vi "CgDataCollect.vi"(0 "Data Queue":refnum<queue>, 1 "Timed Structure Name":string, 2 "Timing Source":string="1 kHz", 5 "VISA resource name":refnum<visa-resource-name>, 7 "Bytes to Read":i32, 9 "Relative Time":u32, 11 "error in (no error)":errorcluster, 12 "Time Loop Priority":i32=100, 13 "Time Bytes Before Output":i16) -> (4 "Queue Out":refnum<queue>, 6 "VISA resource name out":refnum<visa-resource-name>, 8 "Timing Array":u32[](array[numeric]), 15 "error out":errorcluster)   [LabVIEW 2012]
doc: "Collects data from the cyberglove.\nQueries the cyberglove for data and sends the data to a queue to be read by an interpreter running in parallel. Using the relative time and the time bytes before output causes the program to put a time stamp in ms before the output."
uses:
  <vilib>/Platform/TimedLoop/XDataNode/timing_clust.ctl
  <vilib>/Platform/TimedLoop/XDataNode/nitl_modes.ctl
  <vilib>/Platform/TimedLoop/XDataNode/wakeup.ctl
  GlobalVariables.vi
  <vilib>/Platform/TimedLoop/XDataNode/XDataNode.xnode
  <vilib>/Platform/TimedLoop/XDataNode/XDNodeRunTimeDep.lvlib
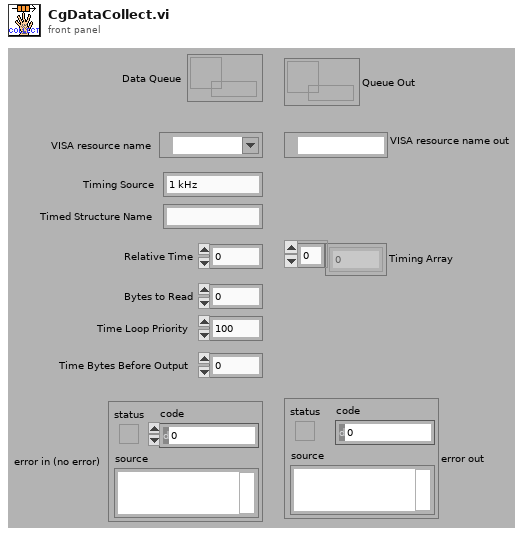
[diagram p1: front panel]
types:
  T1 = typedef "XDNodeRunTimeDep.lvlib/timing_clust.ctl" = cluster{"Expected End [f-1]":u64, "Actual End [f-1]":u64, "Finished Late? [f-1]":bool, "Expected End [i-1]":u64, "Actual End [i-1]":u64, "Finished Late? [i-1]":bool, "Expected Start [i]":u64, "Actual Start [i]":u64, "Expected Start [f]":u64, "Actual Start [f]":u64, "Source Name":string, "Structure Name":string, "Period":i64, "Deadline":i64, "Offset":i64, "Start":i64, "Priority":i32, "Timeout":i32, "Mode":T2, "Wakeup Reason":T3, "Error":errorcluster, "Source Type":string, "Secondary Source Type":string, "Global End Time":u64, "Global Start Time":u64, "Frame Duration":u64, "Iteration Duration":u64, "Assigned CPU":i32, "I/O Scan Engine Mode":u32}
  T2 = typedef "XDNodeRunTimeDep.lvlib/nitl_modes.ctl" = enum32{"No Change", "Process missed periods, maintain original phase", "Discard missed periods, maintain original phase", "Process missed periods, ignore original phase", "Discard missed periods, ignore original phase"}
  T3 = typedef "XDNodeRunTimeDep.lvlib/wakeup.ctl" = enum32{"Normal", "Aborted", "Asynchronous wakeup", "Timing source error", "Timed loop error", "Timeout"}
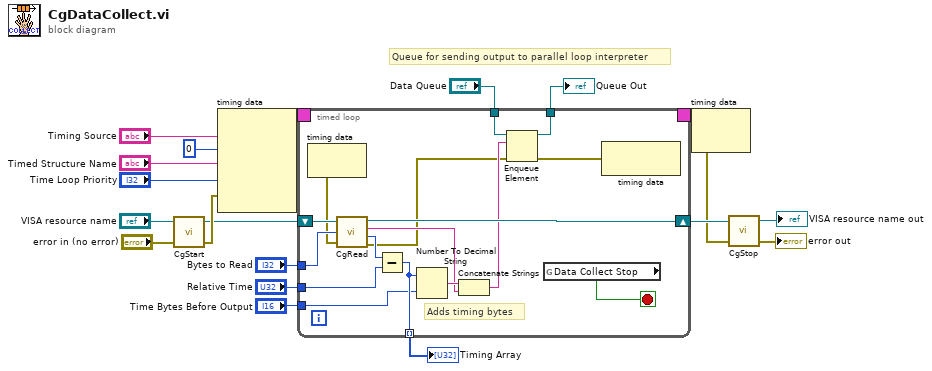
[diagram p0: block diagram]
diagram:
  # "Queue for sending output to parallel loop interpreter"
  n1 = call "CgStart.vi"("error in (no error)"="error in (no error)", "VISA resource name"="VISA resource name") -> ("error out"=w6:errorcluster, "VISA resource name out"=w5:refnum<visa-resource-name>)  [unwired: 2 in]
  n2 = node-c288("Timing Source", i64 0 ("Period"), "Timed Structure Name", "Time Loop Priority", w6) -> (w20:T1)
  n3 = timed-loop {
    timing: w20 -> [_]
    timing-out: [_] -> w19
    tunnel: "Bytes to Read" -> [w35]
    shift-right: [w34] -> w9
    shift-left: w5 -> [w36]
    tunnel: "Data Queue" -> [w33]
    tunnel: [w32] -> w10
    tunnel: "Relative Time" -> [w30]
    tunnel: [w28] -> w3 mode=indexing
    tunnel: "Time Bytes Before Output" -> [w23]
    stop <- w24 stop-if-true
    # "Adds timing bytes"
    n4 = node-c288() -> (w31:errorcluster)  [unwired: 1 in]
    n5 = call "CgRead.vi"("VISA resource name"=w36, "Bytes"=w35, "error in (no error)"=w31) -> ("VISA resource name out"=w34:refnum<visa-resource-name>, "Cyberglove Output"=w26:string, "Time"=w29:u32, "error out"=w22:errorcluster)
    n6 = Subtract(x=w29, y=w30) -> (x-y=w28:u32)
    n7 = Number To Decimal String(number=w28, width (-)=w23) -> (decimal integer string=w27:string)
    n8 = Concatenate Strings(w27, w26) -> (w25:string)
    n9 = Enqueue Element(queue=w33, element=w25, error in (no error)=w22) -> (queue out=w32:refnum<queue>, error out=w21:errorcluster)  [unwired: 1 in, 1 out]
    n10 = global read "GlobalVariables.vi" "Data Collect Stop"() -> (w24:bool)
    n11 = node-c288(w21) -> ()  [unwired: 1 out]
  }
  "Queue Out" <- w10
  "Timing Array" <- w3
  n12 = node-c288(w19) -> (w1:errorcluster)
  n13 = call "CgStop.vi"("error in (no error)"=w1, "VISA resource name"=w9) -> ("error out"=→"error out":errorcluster, "VISA resource name out"=→"VISA resource name out":refnum<visa-resource-name>)  [unwired: 2 in]
